vi "axex_get_sheet_range.vi"(8 "error in":errorcluster, 11 "AX Excel instance in":T1) -> (0 "error out":errorcluster, 1 "columns":i32, 2 "rows":i32, 3 "AX Excel instance out":T1)   [LabVIEW 2020, in "AX Excel.lvlib"]
doc: "Call this to get used range of the sheets (used columns and rows count)."
uses:
  AX Excel.lvlib
  axex_instance.ctl
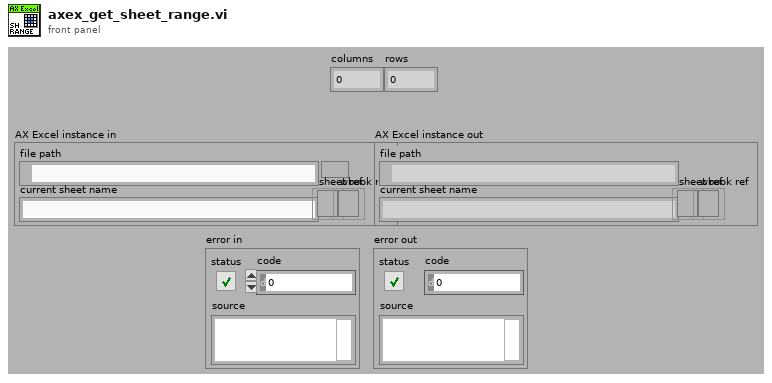
[diagram p1: front panel]
types:
  T1 = typedef "AX Excel.lvlib/axex_instance.ctl" = cluster{"file path":path, "current sheet name":string, "sheet ref":refnum<k7>, "wbook ref":refnum<k7>}
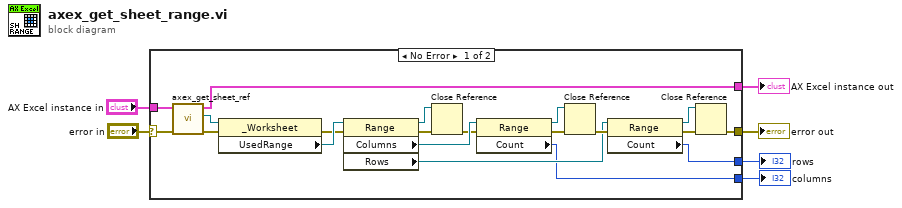
[diagram p0: block diagram]
diagram:
  n1 = case shown="No Error" "error in" {
    selector: "error in" -> [w7 w27]
    tunnel: "AX Excel instance in" -> [w26 w28]
    tunnel: [w25 w28] -> w5
    tunnel: [w11 w27] -> w4
    tunnel: [w10 _] -> w3
    tunnel: [w9 _] -> w2
    frame No Error {
      n2 = call "axex_get_sheet_ref.vi"("error in"=w7, "AX Excel instance in"=w26) -> ("error out"=w24:errorcluster, "sheet ref out"=w23:refnum<k7>, "AX Excel instance out"=w25:T1)  [unwired: 6 in, 1 out]
      n3 = property class="_Worksheet"(reference=w23, error in=w24) -> (error out=w8:errorcluster, "UsedRange"=w22:refnum<k7>)  [unwired: 1 out]
      n4 = property class="Range"(reference=w22, error in=w8) -> (reference out=w19:refnum<k7>, error out=w20:errorcluster, "Columns"=w21:refnum<k7>, "Rows"=w12:refnum<k7>)
      n5 = Close Reference(reference=w19, error in (no error)=w20) -> (error out=w18:errorcluster)
      n6 = property class="Range"(reference=w21, error in=w18) -> (reference out=w16:refnum<k7>, error out=w17:errorcluster, "Count"=w10:i32)
      n7 = Close Reference(reference=w16, error in (no error)=w17) -> (error out=w13:errorcluster)
      n8 = property class="Range"(reference=w12, error in=w13) -> (reference out=w15:refnum<k7>, error out=w14:errorcluster, "Count"=w9:i32)
      n9 = Close Reference(reference=w15, error in (no error)=w14) -> (error out=w11:errorcluster)
    }
    frame Error {
    }
  }
  "error out" <- w4
  "AX Excel instance out" <- w5
  "columns" <- w3
  "rows" <- w2
